vi "FRCts20_WebMethods_Comment_DELETE.vi"(7 "httpRequestID":u32, 10 "comment":string, 11 "request":string) -> ()   [LabVIEW 2014, in "FRCts20_WebMethods.lvlib"]
doc: "<B>DELETE</B> the specified <B>comment</B> resource\n\nhttp://<server address>:<port>/FRCts/request/<B>request</B>/comment/<B>comment</B>\n\n{requires authentication}"
uses:
  FRCts20_WebMethods.lvlib
  <vilib>/wsapi/NI_WebServices.lvlib
  Backend/source/VI Source/FRCts20_Backend_API/FRCts20_Backend_API_Note.ctl
  Backend/source/VI Source/FRCts20_Backend_API/FRCts20_Backend_API_Command_Note.ctl
  Backend/source/VI Source/FRCts20_Backend_API/FRCts20_Backend_API_Comment.vi
panel:
  in  "query":string
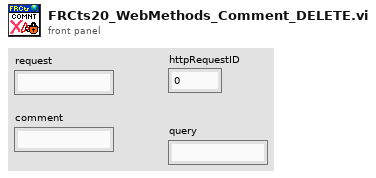
[diagram p1: front panel]
types:
  T1 = typedef "FRCts20_Backend_API.lvlib/FRCts20_Backend_API_Command_Note.ctl" = string
  T2 = typedef "FRCts20_Backend_API.lvlib/FRCts20_Backend_API_Note.ctl" = cluster{"Note Index":u32, "Request Index":u32, "Author":string, "Time Entered":timestamp, "Text":string, "Solution":bool, "APIReturn":string}
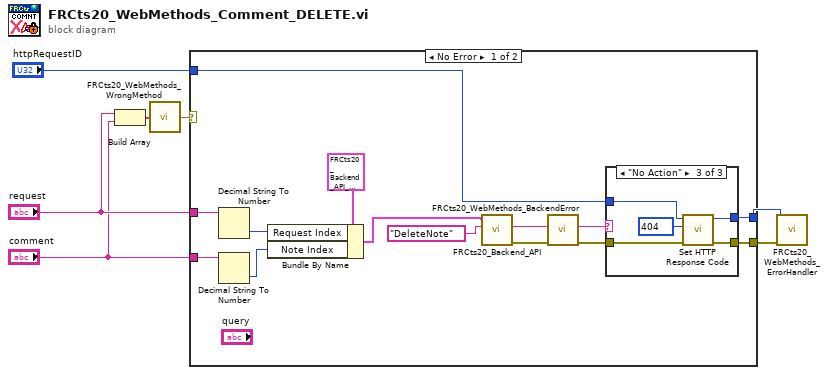
[diagram p0: block diagram]
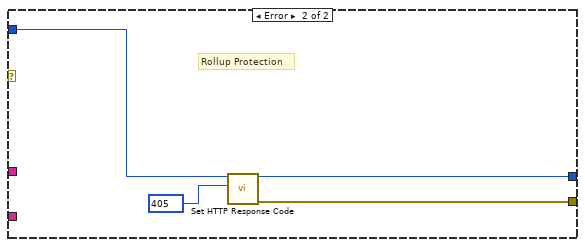
[diagram p4: hidden frame]
diagram:
  n1 = Build Array("request", "comment") -> (w6:string[])
  n2 = call "FRCts20_WebMethods_WrongMethod.vi"(4:w6) -> (1:w7)  [unwired: 3 in, 1 out]
  n3 = case shown="No Error" w7 {
    tunnel: "httpRequestID" -> [w14 w34]
    tunnel: [w13 w32] -> w3
    tunnel: [w12 w31] -> w4
    tunnel: "request" -> [w21 _]
    tunnel: "comment" -> [w20 _]
    frame No Error {
      n4 = Decimal String To Number(string=w21) -> (number=w18:i32)  [unwired: 2 in, 1 out]
      n5 = Decimal String To Number(string=w20) -> (number=w17:i32)  [unwired: 2 in, 1 out]
      n6 = Bundle By Name(cluster=T2 {"Note Index"=0, "Request Index"=0, "Author"="", "Time Entered"=timestamp(0 s since 1904-01-01), "Text"="", "Solution"=FALSE, "APIReturn"=""} ("Note"), "Request Index"=w18, "Note Index"=w17) -> (w9:T2)
      n7 = call-poly "FRCts20_Backend_API.vi"("Command"=T1 "DeleteNote", "Note In"=w9) -> ("error out"=w11:errorcluster, "Status"=w10:string)  [unwired: 7 in, 1 out]
      n8 = call "FRCts20_WebMethods_BackendError.vi"("error in (no error)"=w11, "Status"=w10) -> ("error out"=w15:errorcluster, "Status out"=w16:string)  [unwired: 8 in]
      n9 = case shown="\"No Action\"" w16 {
        tunnel: w15 -> [w22 w24 w27]
        tunnel: w14 -> [w23 w25 w28]
        tunnel: [w23 w25 w29] -> w13
        tunnel: [w22 w24 w30] -> w12
        frame "Backend Error", Default {
        }
        frame "Success" {
        }
        frame "No Action" {
          w26 = 404 items=["100"=100, "101"=101, "200"=200, "201"=201, "202"=202, "203"=203, "204"=204, "205"=205, "206"=206, "300"=300, "301"=301, "302"=302, "303"=303, "304"=304, "305"=305, "306"=306, "307"=307, "400"=400, "401"=401, "402"=402, "403"=403, "404"=404, "405"=405, "406"=406, "407"=407, "408"=408, "409"=409, "410"=410, "411"=411, "412"=412, "413"=413, "414"=414, "415"=415, "416"=416, "417"=417, "500"=500, "501"=501, "502"=502, "503"=503, "504"=504, "505"=505] ("response code (200)")
          n10 = call <vilib>:"Set HTTP Response Code.vi"("error in (no error)"=w27, "response code (200)"=w26, "httpRequestID"=w28) -> ("error out"=w30:errorcluster, "httpRequestID out"=w29:u32)  [unwired: 7 in]
        }
      }
    }
    frame Error {
      w33 = 405 items=["100"=100, "101"=101, "200"=200, "201"=201, "202"=202, "203"=203, "204"=204, "205"=205, "206"=206, "300"=300, "301"=301, "302"=302, "303"=303, "304"=304, "305"=305, "306"=306, "307"=307, "400"=400, "401"=401, "402"=402, "403"=403, "404"=404, "405"=405, "406"=406, "407"=407, "408"=408, "409"=409, "410"=410, "411"=411, "412"=412, "413"=413, "414"=414, "415"=415, "416"=416, "417"=417, "500"=500, "501"=501, "502"=502, "503"=503, "504"=504, "505"=505] ("response code (200)")
      # "Rollup Protection"
      n11 = call <vilib>:"Set HTTP Response Code.vi"("response code (200)"=w33, "httpRequestID"=w34) -> ("error out"=w31:errorcluster, "httpRequestID out"=w32:u32)  [unwired: 8 in]
    }
  }
  n12 = call "FRCts20_WebMethods_ErrorHandler.vi"("error in"=w4, "LabVIEW Web Service Request"=w3) -> ()  [unwired: 8 in, 2 out]
